vi "请求注销.vi"(8 "error in (no error)":errorcluster caption="错误输入（无错误）", 10 "数据采集.lvclass":refnum<class "数据采集.lvclass">, 11 "订阅者接口 输入":refnum<class "订阅者接口.lvclass"> caption="DNL_LabVIEW Object in") -> (0 "error out":errorcluster caption="错误输出", 2 "数据采集.lvclass":refnum<class "数据采集.lvclass">, 3 "订阅者接口 输出":refnum<class "订阅者接口.lvclass"> caption="DNL_LabVIEW Object out")   [LabVIEW 2013, in "订阅者接口.lvclass"]
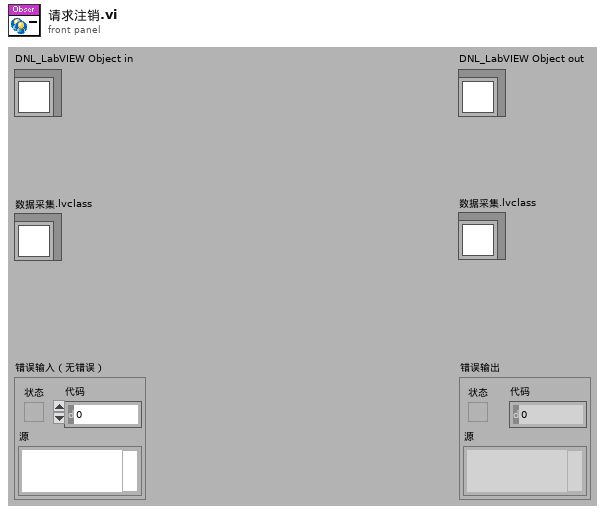
[diagram p1: front panel]
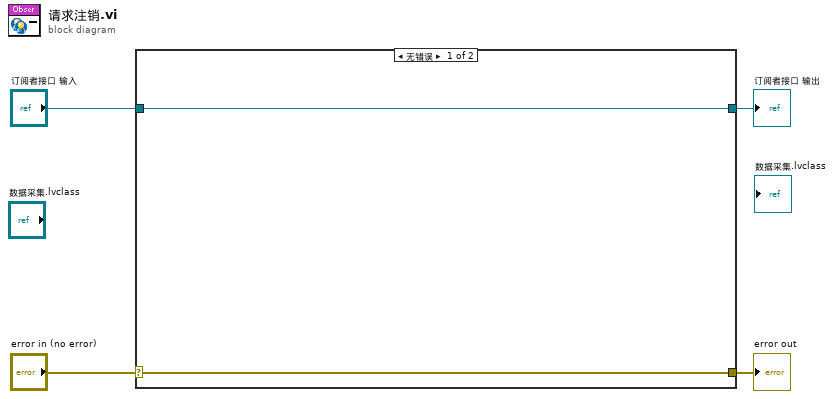
[diagram p0: block diagram]
diagram:
  n1 = case shown="无错误" "error in (no error)" {
    selector: "error in (no error)" -> [w5 w8]
    tunnel: [w5 w8] -> w3
    tunnel: [w6 w7] -> w1
    tunnel: "订阅者接口 输入" -> [w6 w7]
    frame No Error {
    }
    frame Error {
    }
  }
  "error out" <- w3
  "订阅者接口 输出" <- w1
